vi "cargame.vi"(11 "NXT/EV3":T1) -> (3 "NXT/EV3 2":T1)   [LabVIEW 2013]
uses:
  <vilib>/NXT/Subs/LVHSConnector.ctl
  <vilib>/NXT/LegoClasses/BrickReference/BrickReference.lvclass
  <vilib>/NXT/Dual Mode Library/Display/clearDisplay.vi
  <vilib>/NXT/Dual Mode Library/Display/drawPicture.vi
  <vilib>/NXT/Dual Mode Library/Advanced/NXTFlag_Get_Integer.vi
  <vilib>/NXT/Dual Mode Library/Motors/Rotation.vi
  <vilib>/NXT/Dual Mode Library/prims/inRangeAndCoerce/inRangeAndCoerce_int.vi
  <vilib>/NXT/Dual Mode Library/Waits/Wait_Num.vi
  <vilib>/NXT/Dual Mode Library/Display/eraseRect.vi
  <vilib>/NXT/Dual Mode Library/Display/drawRect_filled.vi
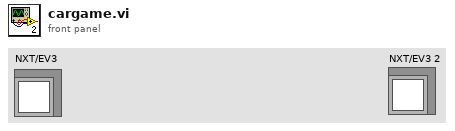
[diagram p1: front panel]
types:
  T1 = typedef "LVHSConnector.ctl" = refnum<class "BrickReference.lvclass">
  T2 = cluster{"upper limit":i32, "upper limit":i32, "upper limit":i32, "upper limit":i32}
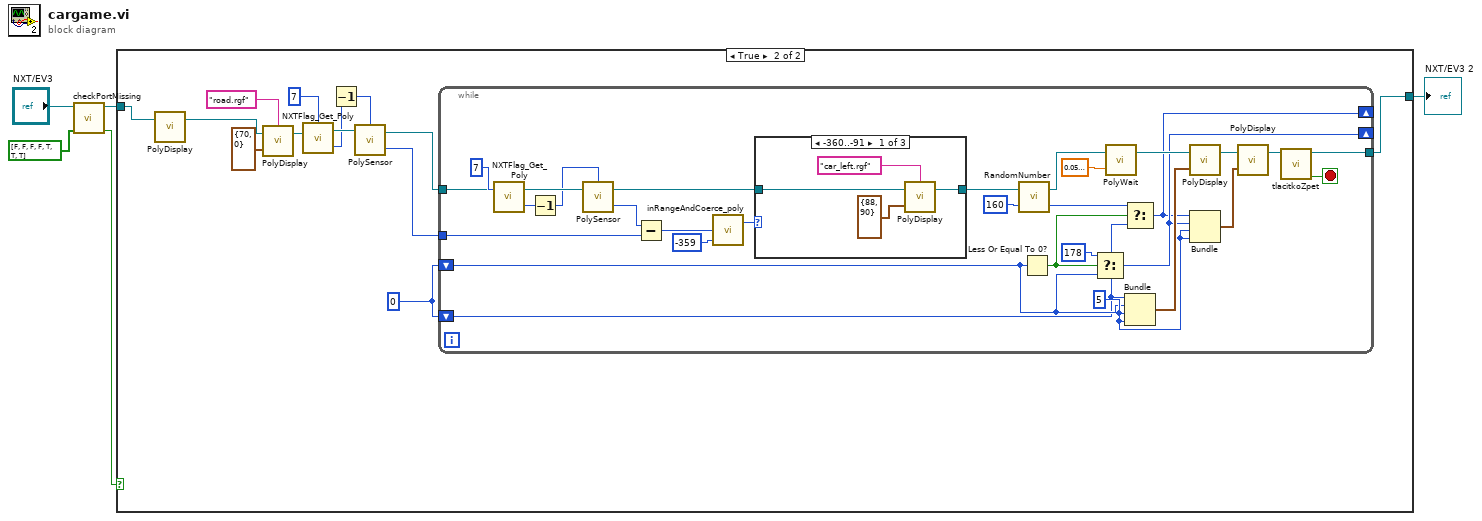
[diagram p0: block diagram]
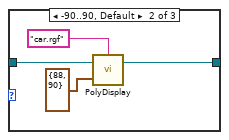
[diagram p3: hidden frame]
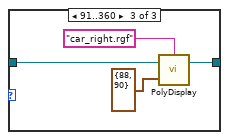
[diagram p4: hidden frame]
diagram:
  n1 = call "checkPortMissing.vi"("Required"=bool[] [FALSE, FALSE, FALSE, FALSE, TRUE, TRUE, TRUE], "NXT/EV3"="NXT/EV3") -> ("Success"=w3:bool, "NXT/EV3"=w1:T1)  [unwired: 8 in]
  n2 = case shown="True" w3 {
    tunnel: [w6 w10] -> w2
    tunnel: w1 -> [w6 w8]
    frame False {
      # "Controllers unavailable"
    }
    frame True {
      w7 = 0 ("upper limit")
      n3 = call-poly <vilib>:"PolyDisplay.vi"("NXT/EV3"=w8) -> ("NXT/EV3"=w9:T1)  [unwired: 3 in]
      n4 = call-poly <vilib>:"PolyDisplay.vi"("Origin"=cluster{"X":i16, "Y":i16} {"X"=70, "Y"=0}, "NXT/EV3"=w9, "Filename (*.ric/*.rgf)"="road.rgf") -> ("NXT/EV3"=w11:T1)  [unwired: 1 in]
      n5 = call-poly <vilib>:"NXTFlag_Get_Poly.vi"("NXT/EV3"=w11, "NXT/EV3 Flag Number"=7) -> ("Flag Value"=w17:i32, "NXT/EV3"=w19:T1)  [unwired: 1 in]
      n6 = Decrement(x=w17) -> (x-1=w16:i32)
      n7 = call-poly <vilib>:"PolySensor.vi"("NXT/EV3"=w19, "Port (Port A)"=w16) -> ("Angle of Rotation"=w14:i32, "NXT/EV3"=w15:T1)  [unwired: 1 in]
      n8 = while {
        tunnel: w15 -> [w45]
        tunnel: w14 -> [w43]
        tunnel: [w22] -> w10
        shift-right: [w27] -> _
        shift-left: w7 -> [w29]
        shift-right: [w28] -> _
        shift-left: w7 -> [w32]
        stop <- w20 stop-if-true
        w33 = 5 ("upper limit")
        n9 = call-poly <vilib>:"NXTFlag_Get_Poly.vi"("NXT/EV3"=w45, "NXT/EV3 Flag Number"=7) -> ("Flag Value"=w47:i32, "NXT/EV3"=w49:T1)  [unwired: 1 in]
        n10 = Decrement(x=w47) -> (x-1=w46:i32)
        n11 = call-poly <vilib>:"PolySensor.vi"("NXT/EV3"=w49, "Port (Port A)"=w46) -> ("Angle of Rotation"=w44:i32, "NXT/EV3"=w41:T1)  [unwired: 1 in]
        n12 = Subtract(x=w44, y=w43) -> (x-y=w40:i32)
        n13 = call-poly <vilib>:"inRangeAndCoerce_poly.vi"("lower limit"=-359, "x"=w40) -> ("coerced(x)"=w39:i32)  [unwired: 1 in, 1 out]
        n14 = case shown="-360..-91" w39 {
          tunnel: [w50 w55 w58] -> w24
          tunnel: w41 -> [w51 w54 w59]
          frame -360..-91 {
            n15 = call-poly <vilib>:"PolyDisplay.vi"("Origin"=cluster{"X":i16, "Y":i16} {"X"=88, "Y"=90}, "NXT/EV3"=w51, "Filename (*.ric/*.rgf)"="car_left.rgf") -> ("NXT/EV3"=w50:T1)  [unwired: 1 in]
          }
          frame -90..90, Default {
            n16 = call-poly <vilib>:"PolyDisplay.vi"("Origin"=cluster{"X":i16, "Y":i16} {"X"=88, "Y"=90}, "NXT/EV3"=w54, "Filename (*.ric/*.rgf)"="car.rgf") -> ("NXT/EV3"=w55:T1)  [unwired: 1 in]
          }
          frame 91..360 {
            n17 = call-poly <vilib>:"PolyDisplay.vi"("Origin"=cluster{"X":i16, "Y":i16} {"X"=88, "Y"=90}, "NXT/EV3"=w59, "Filename (*.ric/*.rgf)"="car_right.rgf") -> ("NXT/EV3"=w58:T1)  [unwired: 1 in]
          }
        }
        n18 = call <vilib>:"RandomNumber.vi"("Max Value"=u16 160, "NXT"=w24) -> ("Random Number"=w25:u16, "NXT"=w23:T1)  [unwired: 1 in]
        n19 = Less Or Equal To 0?(x=w32) -> (x <= 0?=w30:bool)
        n20 = Select(t=178, s=w30, f=w32) -> (s? t:f=w28:i32)
        n21 = call-poly <vilib>:"PolyWait.vi"("Time (1 sec)"=sgl 0.05, "NXT/EV3"=w23) -> ("NXT/EV3"=w36:T1)  [unwired: 2 in]
        n22 = Select(t=w25, s=w30, f=w29) -> (s? t:f=w27:i32)
        n23 = Bundle("upper limit"=w29, "upper limit"=w32, "upper limit"=w33, "upper limit"=w33) -> (w35:T2)  [unwired: 1 in]
        n24 = call-poly <vilib>:"PolyDisplay.vi"("Rect Parameters"=w35, "NXT/EV3"=w36) -> ("NXT/EV3"=w37:T1)  [unwired: 2 in]
        n25 = Bundle("upper limit"=w27, "upper limit"=w28, "upper limit"=w33, "upper limit"=w33) -> (w34:T2)  [unwired: 1 in]
        n26 = call-poly <vilib>:"PolyDisplay.vi"("Rect Parameters"=w34, "NXT/EV3"=w37) -> ("NXT/EV3"=w21:T1)  [unwired: 2 in]
        n27 = call "tlacitkoZpet.vi"("NXT/EV3"=w21) -> ("Boolean"=w20:bool, "NXT/EV3 2"=w22:T1)  [unwired: 9 in]
      }
    }
  }
  "NXT/EV3 2" <- w2
